vi "HEWH_Emerson_WaterFlowMeter.vi"(8 "error in":errorcluster, 11 "Message Queues out":T2) -> (0 "error out":errorcluster)   [LabVIEW 2023]
uses:
  Tenney/support/Message Queue/All Message Queues.ctl
  Tenney/support/Message Queue/Message Cluster.ctl
  Drivers/Emerson 5700 Transmitter/Type Definitions/Emerson 5700 Data.ctl
  Drivers/Emerson 5700 Transmitter/Type Definitions/Emerson 5700 Modbus Write Coils.ctl
  <vilib>/NI/Modbus Library/API/Wrapper/Create TCP Master.vi
  FVIR and LDO/support/Message Queue/Enqueue Message (Single).vi
  <vilib>/NI/Modbus Library/API/Master/Modbus Master.lvclass
  FVIR and LDO/support/Message Queue/Message Queue.lvlib
  <vilib>/NI/Modbus Library/API/Wrapper/API Main.lvlib
  Tenney/support/Message Queue/Tenney Message Queue.lvlib
panel:
  out "Loop Count":i32
  out "Emerson Flow Meter Data Output":T1
  in  "Debug":bool
  out "Debug":string[](array[string])
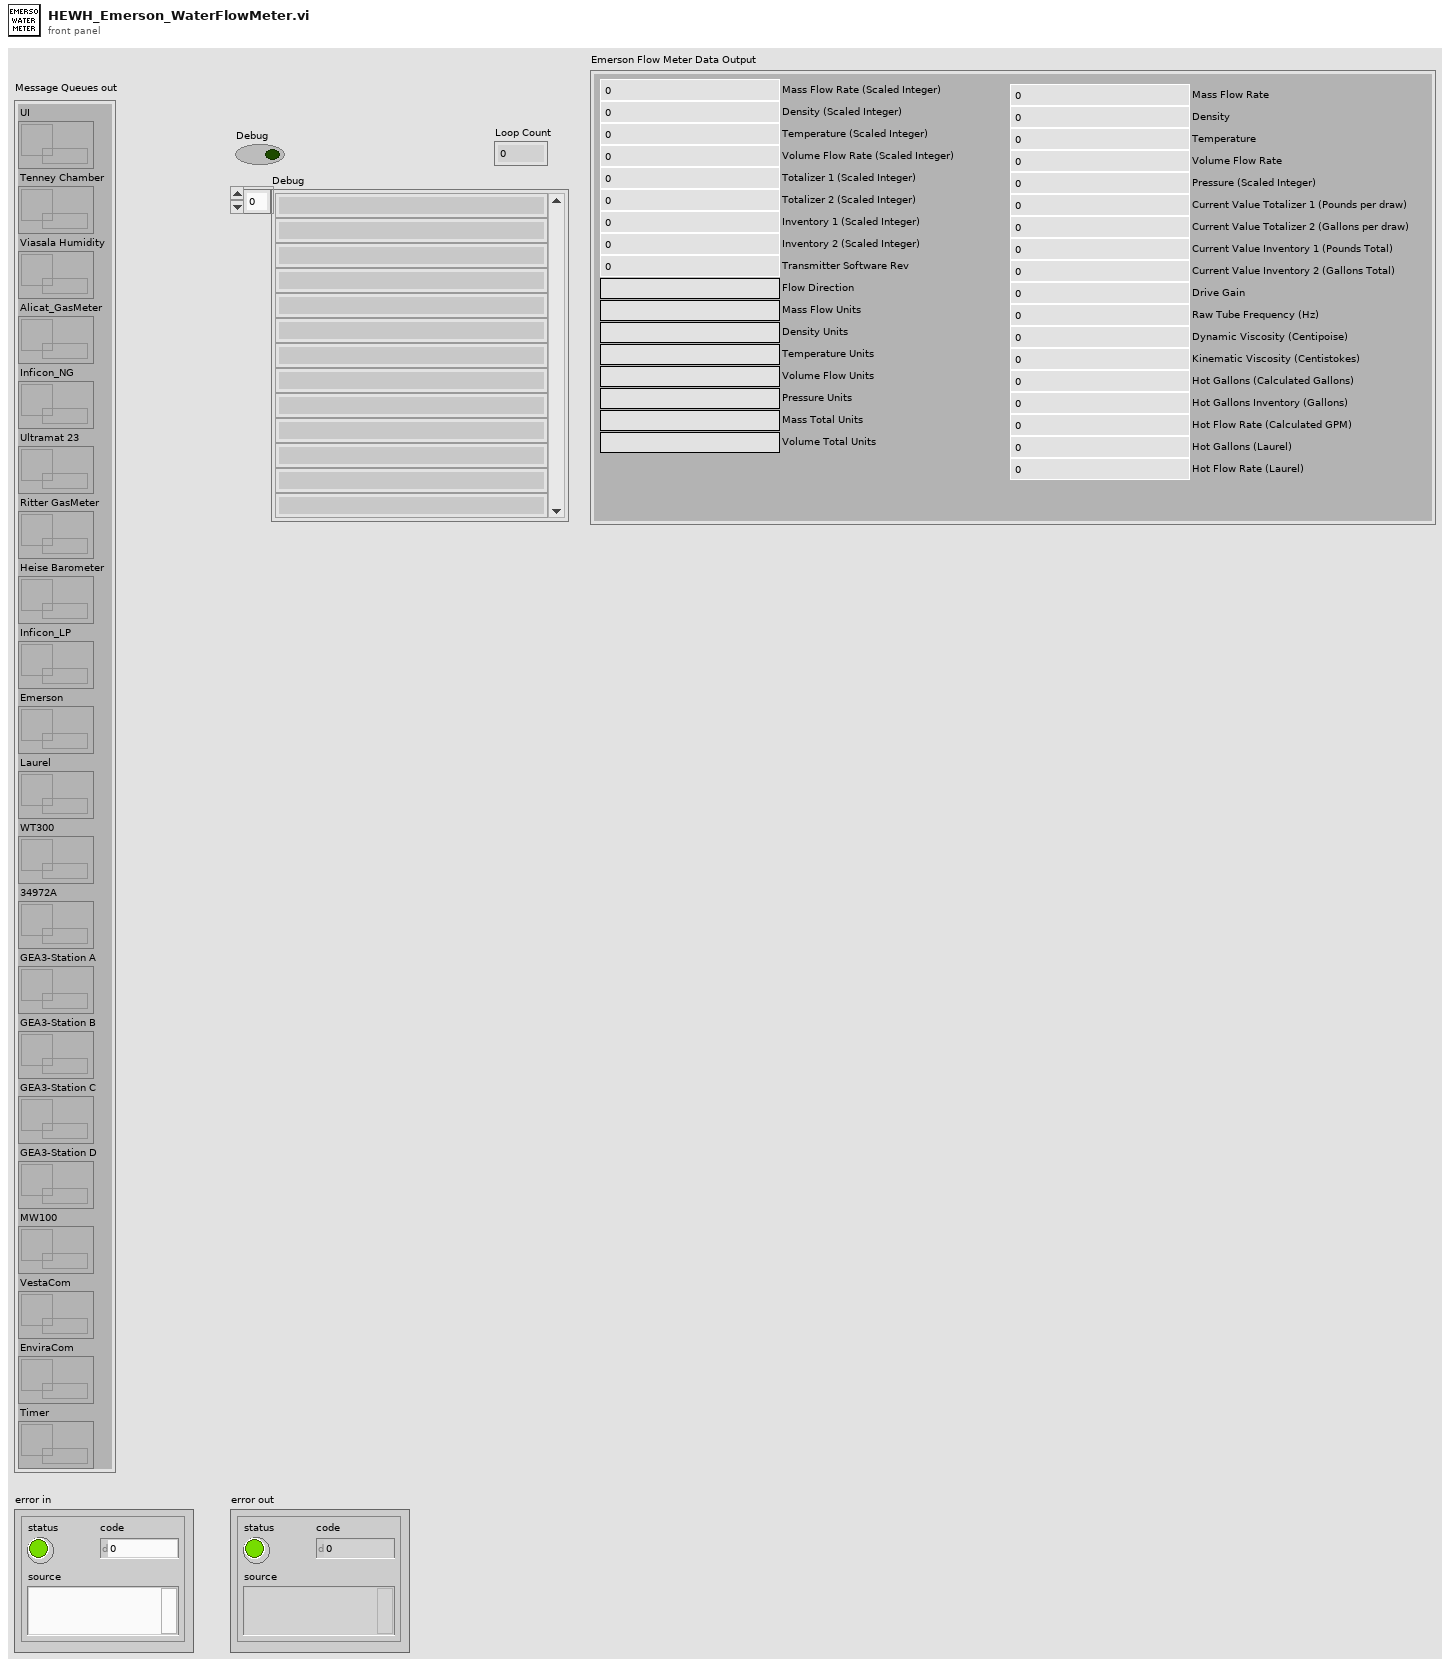
[diagram p1: front panel]
types:
  T1 = typedef "Emerson 5700 Data.ctl" = cluster{"Mass Flow Rate (Scaled Integer)":u16, "Density (Scaled Integer)":u16, "Temperature (Scaled Integer)":u16, "Volume Flow Rate (Scaled Integer)":u16, "Totalizer 1 (Scaled Integer)":u16, "Totalizer 2 (Scaled Integer)":u16, "Transmitter Software Rev":u16, "Flow Direction":string, "Mass Flow Units":string, "Density Units":string, "Temperature Units":string, "Volume Flow Units":string, "Pressure Units":string, "Mass Total Units":string, "Volume Total Units":string, "Inventory 1 (Scaled Integer)":u16, "Inventory 2 (Scaled Integer)":u16, "Mass Flow Rate":dbl, "Density":dbl, "Temperature":dbl, "Volume Flow Rate":dbl, "Pressure (Scaled Integer)":u16, "Current Value Totalizer 1 (Pounds per draw)":dbl, "Current Value Totalizer 2 (Gallons per draw)":dbl, "Current Value Inventory 1 (Pounds Total)":dbl, "Current Value Inventory 2 (Gallons Total)":dbl, "Drive Gain":dbl, "Raw Tube Frequency (Hz)":dbl, "Dynamic Viscosity (Centipoise)":dbl, "Kinematic Viscosity (Centistokes)":dbl, "Hot Gallons (Calculated Gallons)":dbl, "Hot Flow Rate (Calculated GPM)":dbl, "Hot Gallons Inventory (Gallons)":dbl, "Hot Flow Rate (Laurel)":dbl, "Hot Gallons (Laurel)":dbl}
  T2 = typedef "Tenney Message Queue.lvlib/All Message Queues.ctl" = cluster{"UI":refnum<queue>, "Tenney Chamber":refnum<queue>, "Viasala Humidity":refnum<queue>, "Alicat_GasMeter":refnum<queue>, "Inficon_NG":refnum<queue>, "Ultramat 23":refnum<queue>, "Ritter GasMeter":refnum<queue>, "Heise Barometer":refnum<queue>, "Inficon_LP":refnum<queue>, "Emerson":refnum<queue>, "Laurel":refnum<queue>, "WT300":refnum<queue>, "34972A":refnum<queue>, "GEA3-Station A":refnum<queue>, "GEA3-Station B":refnum<queue>, "GEA3-Station C":refnum<queue>, "GEA3-Station D":refnum<queue>, "MW100":refnum<queue>, "VestaCom":refnum<queue>, "EnviraCom":refnum<queue>, "Timer":refnum<queue>}
  T3 = typedef "Emerson 5700 Modbus Write Coils.ctl" = u16
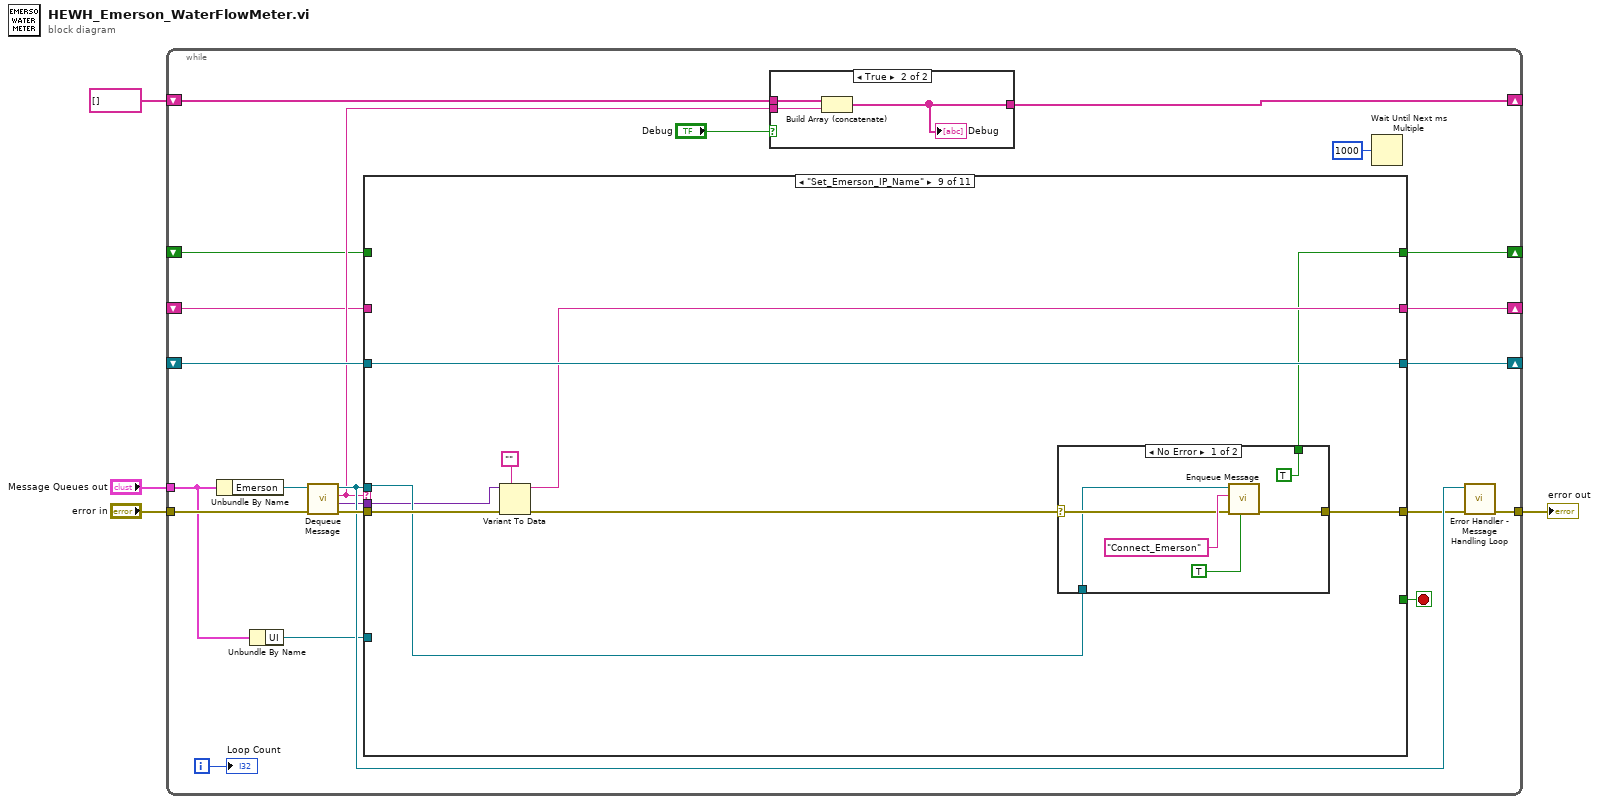
[diagram p0: block diagram]
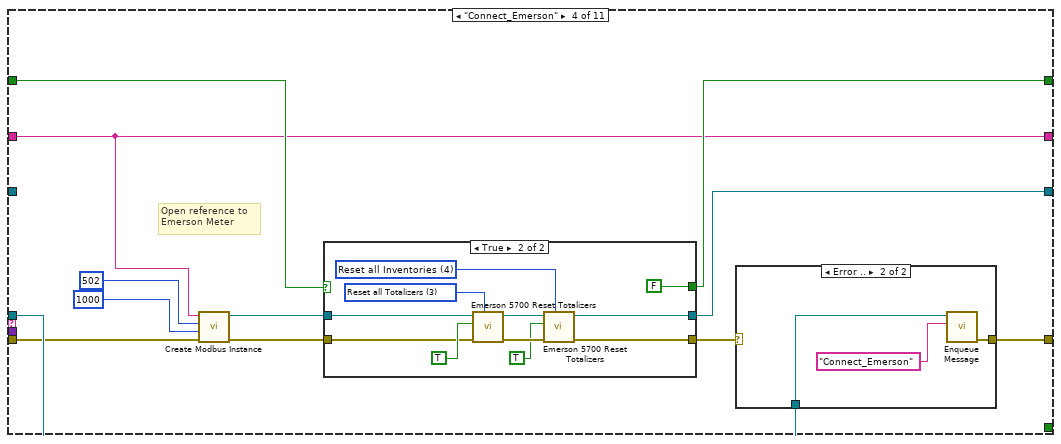
[diagram p6: hidden frame]
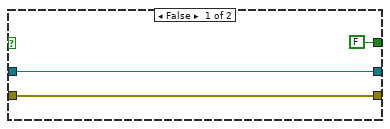
[diagram p7: hidden frame]
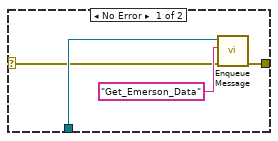
[diagram p8: hidden frame]
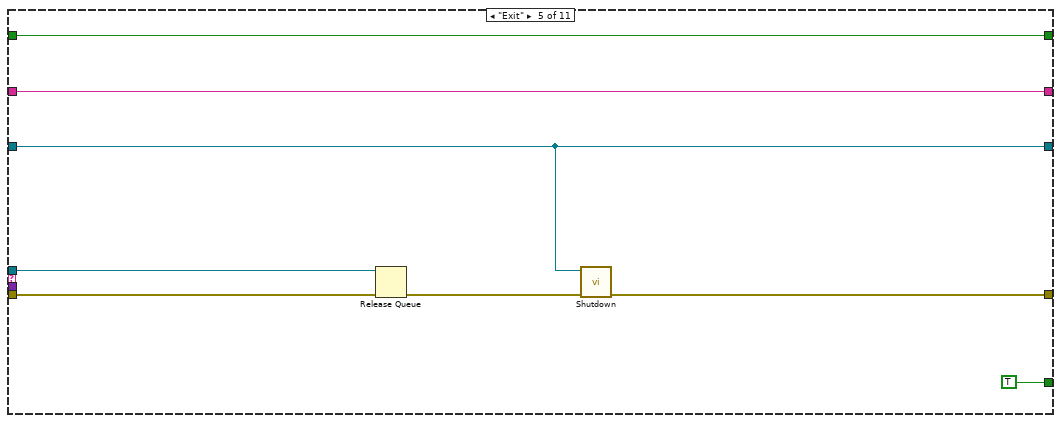
[diagram p9: hidden frame]
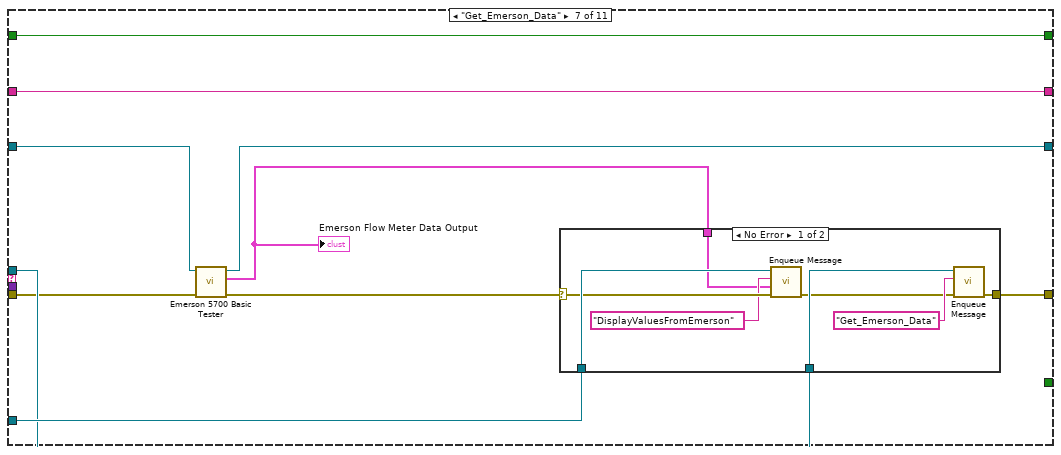
[diagram p11: hidden frame]
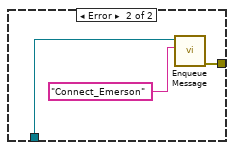
[diagram p12: hidden frame]
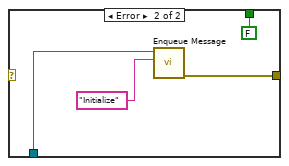
[diagram p14: hidden frame]
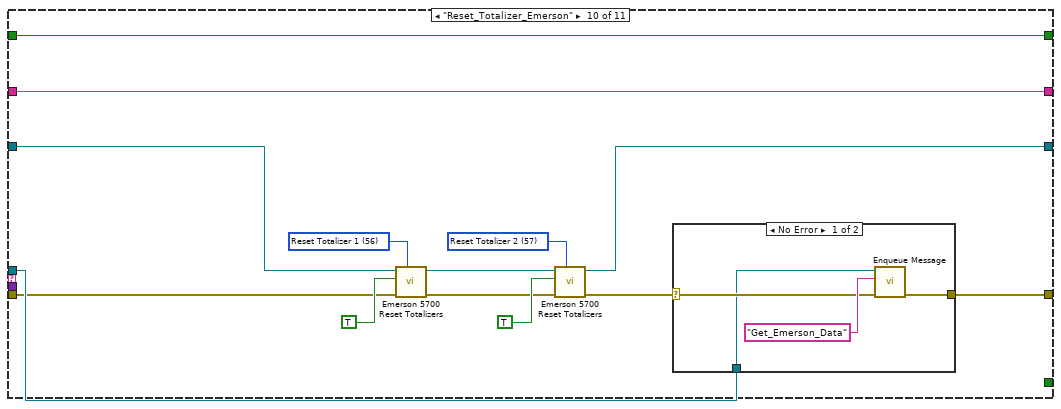
[diagram p15: hidden frame]
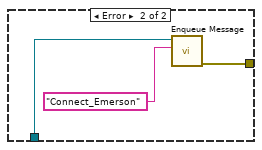
[diagram p16: hidden frame]
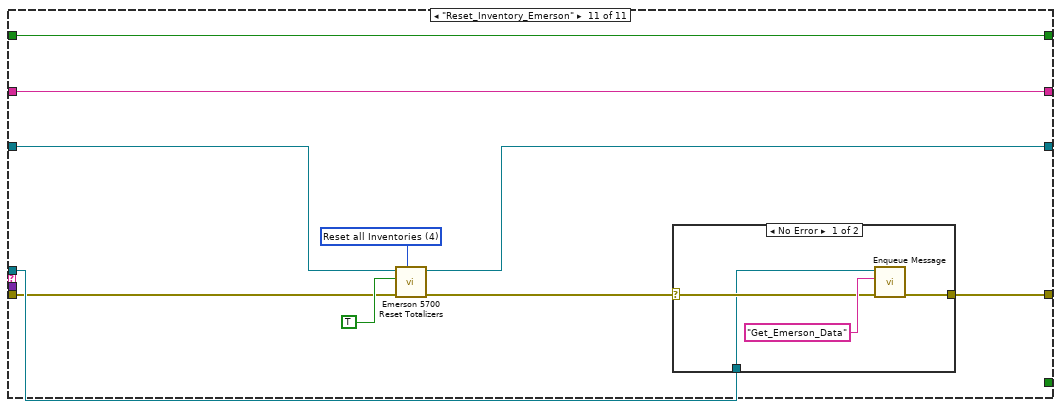
[diagram p17: hidden frame]
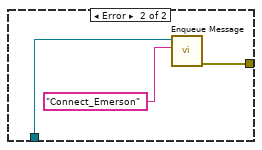
[diagram p18: hidden frame]
diagram:
  n1 = while {
    tunnel: "Message Queues out" -> [w16]
    tunnel: "error in" -> [w25]
    tunnel: [w21] -> w3
    shift-right: [w19] -> _
    shift-left: _ -> [w18]
    shift-right: [w12] -> _
    shift-left: string[] [] -> [w13]
    shift-right: [w10] -> _
    shift-left: _ -> [w9]
    shift-right: [w7] -> _
    shift-left: _ -> [w6]
    i -> [w5]
    stop <- w23 stop-if-true
    n2 = Unbundle By Name(w16) -> ("Emerson"=w26:refnum<queue>)
    n3 = Unbundle By Name(w16) -> ("UI"=w15:refnum<queue>)
    n4 = call "Dequeue Message.vi"("error in (no error)"=w25, "Message Queue"=w26) -> ("error out"=w24:errorcluster, "Message Data"=w8:variant, "Message"=w14:string, "dup Message Queue"=w22:refnum<queue>)  [unwired: 6 in]
    n5 = case shown="\"Set_Emerson_IP_Name\"" w14 {
      tunnel: w24 -> [w33 w35 w40 w50 w77 w86 w94 w111 w119 w136 w157]
      tunnel: [w33 w35 w40 w54 w80 w86 w96 w111 w118 w145 w162] -> w20
      tunnel: [_ _ _ _ TRUE _ _ _ _ _ _] -> w23
      tunnel: w22 -> [_ _ _ w53 w82 _ w95 _ w116 w144 w161]
      tunnel: [w34 w38 w42 w44 w79 w87 w91 w112 w121 w133 w154] -> w19
      tunnel: w18 -> [w34 w38 w42 _ w79 w87 w92 w112 w121 w135 w156]
      tunnel: w15 -> [_ _ _ _ _ _ w97 _ _ _ _]
      tunnel: [w32 w37 w39 w46 w78 w85 w89 w110 w113 w143 w160] -> w10
      tunnel: w9 -> [w32 w37 w39 w47 w78 w85 w89 w110 _ w143 w160]
      tunnel: w8 -> [_ _ _ _ _ _ _ _ w115 _ _]
      tunnel: [w31 w36 w41 w43 w76 w84 w88 w109 w114 w132 w153] -> w7
      tunnel: w6 -> [w31 w36 w41 w43 w76 w84 w88 w109 _ w132 w153]
      frame "---------- Setup ----------" {
      }
      frame Default {
      }
      frame "Initialize" {
      }
      frame "Connect_Emerson" {
        # "Open reference to \nEmerson Meter"
        n6 = call-poly <vilib>:"Create Modbus Instance.vi"("error in"=w50, "connect timeout ms"=1000, "port (502)"=u16 502, "address"=w43) -> ("error out"=w49:errorcluster, "TCP master instance"=w48:refnum<class "Modbus Master.lvclass">)  [unwired: 6 in]
        n7 = case shown="True" w47 {
          tunnel: w49 -> [w56 w62]
          tunnel: [w56 w61] -> w45
          tunnel: w48 -> [w55 w60]
          tunnel: [FALSE FALSE] -> w46
          tunnel: [w55 w58] -> w44
          frame False {
          }
          frame True {
            w66 = T3 4 items=["Start/Stop Inventory 1"=367, "Start/Stop Inventory 2"=368, "Start/Stop all Totalizers and Inventories"=2, "Reset all Totalizers"=3, "Reset all Inventories"=4, "Reset Totalizer 1"=56, "Reset Totalizer 2"=57] ("Reset all Totalizers. 2")
            w64 = T3 3 items=["Start/Stop Inventory 1"=367, "Start/Stop Inventory 2"=368, "Start/Stop all Totalizers and Inventories"=2, "Reset all Totalizers"=3, "Reset all Inventories"=4, "Reset Totalizer 1"=56, "Reset Totalizer 2"=57] ("Reset all Totalizers. 2")
            n8 = call "Emerson 5700 Reset Totalizers.vi"("Reset all Totalizers"=w64, "Error In"=w62, "Coil"=TRUE, "Modbus master in"=w60) -> ("Error Out"=w68:errorcluster, "Modbus master out"=w67:refnum<class "Modbus Master.lvclass">)  [unwired: 6 in]
            n9 = call "Emerson 5700 Reset Totalizers.vi"("Reset all Totalizers"=w66, "Error In"=w68, "Coil"=TRUE, "Modbus master in"=w67) -> ("Error Out"=w61:errorcluster, "Modbus master out"=w58:refnum<class "Modbus Master.lvclass">)  [unwired: 6 in]
          }
        }
        n10 = case shown="Error .." w45 {
          selector: w45 -> [w69 _]
          tunnel: [w71 w74] -> w54
          tunnel: w53 -> [w70 w73]
          frame No Error {
            n11 = call-poly "Enqueue Message.vi"("error in (no error)"=w69, "Message"="Get_Emerson_Data", "Message Queue"=w70) -> ("error out"=w71:errorcluster)  [unwired: 7 in, 1 out]
          }
          frame Error {
            n12 = call-poly "Enqueue Message.vi"("Message"="Connect_Emerson", "Message Queue"=w73) -> ("error out"=w74:errorcluster)  [unwired: 8 in, 1 out]
          }
        }
      }
      frame "Exit" {
        n13 = Release Queue(queue=w82, error in (no error)=w77) -> (error out=w81:errorcluster)  [unwired: 1 in, 2 out]
        n14 = call-dynamic "Shutdown.vi"("error in"=w81, "Modbus master in"=w79) -> ("error out"=w80:errorcluster)  [unwired: 9 in]
      }
      frame "---------- Data Collection ----------" {
      }
      frame "Get_Emerson_Data" {
        n15 = call "Emerson 5700 Basic Tester.vi"("Error In"=w94, "Modbus Master in"=w92) -> ("Error Out"=w93:errorcluster, "Emerson Flow Meter Data Output"=w90:T1, "Modbus master out"=w91:refnum<class "Modbus Master.lvclass">)  [unwired: 7 in]
        "Emerson Flow Meter Data Output" <- w90
        n16 = case shown="No Error" w93 {
          selector: w93 -> [w100 _]
          tunnel: w97 -> [w105 _]
          tunnel: [w104 w107] -> w96
          tunnel: w95 -> [w103 w106]
          tunnel: w90 -> [w98 _]
          frame No Error {
            n17 = call-poly "Enqueue Message.vi"("error in (no error)"=w100, "Message Data"=w98, "Message"="DisplayValuesFromEmerson", "Message Queue"=w105) -> ("error out"=w101:errorcluster)  [unwired: 6 in, 1 out]
            n18 = call-poly "Enqueue Message.vi"("error in (no error)"=w101, "Message"="Get_Emerson_Data", "Message Queue"=w103) -> ("error out"=w104:errorcluster)  [unwired: 7 in, 1 out]
          }
          frame Error {
            n19 = call-poly "Enqueue Message.vi"("Message"="Connect_Emerson", "Message Queue"=w106) -> ("error out"=w107:errorcluster)  [unwired: 8 in, 1 out]
          }
        }
      }
      frame "---------- Events ----------" {
      }
      frame "Set_Emerson_IP_Name" {
        n20 = Variant To Data(error in=w119, type="", Variant=w115) -> (data=w114:string, error out=w117:errorcluster)
        n21 = case shown="No Error" w117 {
          selector: w117 -> [w125 _]
          tunnel: [w124 w130] -> w118
          tunnel: w116 -> [w123 w129]
          tunnel: [TRUE FALSE] -> w113
          frame No Error {
            n22 = call-poly "Enqueue Message.vi"("Priority Message? (F)"=TRUE, "error in (no error)"=w125, "Message"="Connect_Emerson", "Message Queue"=w123) -> ("error out"=w124:errorcluster)  [unwired: 6 in, 1 out]
          }
          frame Error {
            n23 = call-poly "Enqueue Message.vi"("Message"="Initialize", "Message Queue"=w129) -> ("error out"=w130:errorcluster)  [unwired: 8 in, 1 out]
          }
        }
      }
      frame "Reset_Totalizer_Emerson" {
        w139 = T3 57 items=["Start/Stop Inventory 1"=367, "Start/Stop Inventory 2"=368, "Start/Stop all Totalizers and Inventories"=2, "Reset all Totalizers"=3, "Reset all Inventories"=4, "Reset Totalizer 1"=56, "Reset Totalizer 2"=57] ("Reset all Totalizers. 2")
        w142 = T3 56 items=["Start/Stop Inventory 1"=367, "Start/Stop Inventory 2"=368, "Start/Stop all Totalizers and Inventories"=2, "Reset all Totalizers"=3, "Reset all Inventories"=4, "Reset Totalizer 1"=56, "Reset Totalizer 2"=57] ("Reset all Totalizers. 2")
        n24 = call "Emerson 5700 Reset Totalizers.vi"("Reset all Totalizers"=w142, "Error In"=w136, "Coil"=TRUE, "Modbus master in"=w135) -> ("Error Out"=w138:errorcluster, "Modbus master out"=w134:refnum<class "Modbus Master.lvclass">)  [unwired: 6 in]
        n25 = call "Emerson 5700 Reset Totalizers.vi"("Reset all Totalizers"=w139, "Error In"=w138, "Coil"=TRUE, "Modbus master in"=w134) -> ("Error Out"=w137:errorcluster, "Modbus master out"=w133:refnum<class "Modbus Master.lvclass">)  [unwired: 6 in]
        n26 = case shown="No Error" w137 {
          selector: w137 -> [w148 _]
          tunnel: [w147 w151] -> w145
          tunnel: w144 -> [w146 w150]
          frame No Error {
            n27 = call-poly "Enqueue Message.vi"("error in (no error)"=w148, "Message"="Get_Emerson_Data", "Message Queue"=w146) -> ("error out"=w147:errorcluster)  [unwired: 7 in, 1 out]
          }
          frame Error {
            n28 = call-poly "Enqueue Message.vi"("Message"="Connect_Emerson", "Message Queue"=w150) -> ("error out"=w151:errorcluster)  [unwired: 8 in, 1 out]
          }
        }
      }
      frame "Reset_Inventory_Emerson" {
        w159 = T3 4 items=["Start/Stop Inventory 1"=367, "Start/Stop Inventory 2"=368, "Start/Stop all Totalizers and Inventories"=2, "Reset all Totalizers"=3, "Reset all Inventories"=4, "Reset Totalizer 1"=56, "Reset Totalizer 2"=57] ("Reset all Totalizers. 2")
        n29 = call "Emerson 5700 Reset Totalizers.vi"("Reset all Totalizers"=w159, "Error In"=w157, "Coil"=TRUE, "Modbus master in"=w156) -> ("Error Out"=w155:errorcluster, "Modbus master out"=w154:refnum<class "Modbus Master.lvclass">)  [unwired: 6 in]
        n30 = case shown="No Error" w155 {
          selector: w155 -> [w165 _]
          tunnel: [w164 w168] -> w162
          tunnel: w161 -> [w163 w167]
          frame No Error {
            n31 = call-poly "Enqueue Message.vi"("error in (no error)"=w165, "Message"="Get_Emerson_Data", "Message Queue"=w163) -> ("error out"=w164:errorcluster)  [unwired: 7 in, 1 out]
          }
          frame Error {
            n32 = call-poly "Enqueue Message.vi"("Message"="Connect_Emerson", "Message Queue"=w167) -> ("error out"=w168:errorcluster)  [unwired: 8 in, 1 out]
          }
        }
      }
    }
    n33 = case shown="True" "Debug" {
      tunnel: w14 -> [_ w30]
      tunnel: w13 -> [w27 w29]
      tunnel: [w27 w28] -> w12
      frame False {
      }
      frame True {
        n34 = Build Array (concatenate)(w29, w30) -> (w28:string[])
        "Debug" <- w28
      }
    }
    n35 = Wait Until Next ms Multiple(millisecond multiple=u32 1000) -> ()  [unwired: 1 out]
    n36 = call "Error Handler - Message Handling Loop.vi"("error in (no error)"=w20, "Message Queue"=w22) -> ("dup error in"=w21:errorcluster)  [unwired: 8 in, 1 out]
    "Loop Count" <- w5
  }
  "error out" <- w3
